vi "Parcial-Ascensor.vi"() -> ()   [LabVIEW 2018]
panel:
  out "PISO 4":bool
  out "PISO 3":bool
  out "PISO 2":bool
  out "PISO 1":bool
  in  "Ring":u16(ring)
  in  "Bajar4":bool
  in  "Bajar3":bool
  in  "Subir3":bool
  in  "Bajar2":bool
  in  "Subir2":bool
  in  "Subir1":bool
  out "4":bool
  out "3":bool
  out "2":bool
  out "1":bool
  out "P-der":dbl(slide) scale=0.0..10.0
  out "P-izq":dbl(slide)
  in  "Cerrar":bool
  in  "Abrir":bool
  out "Ascensor":bool
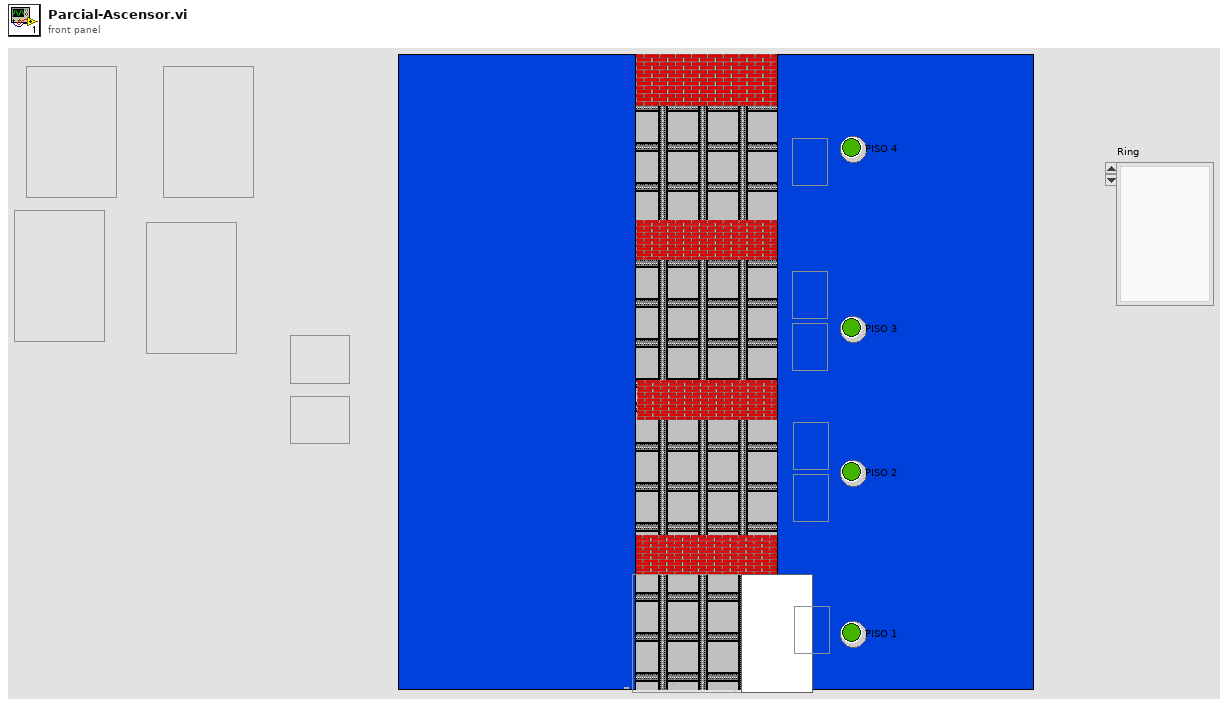
[diagram p1: front panel]
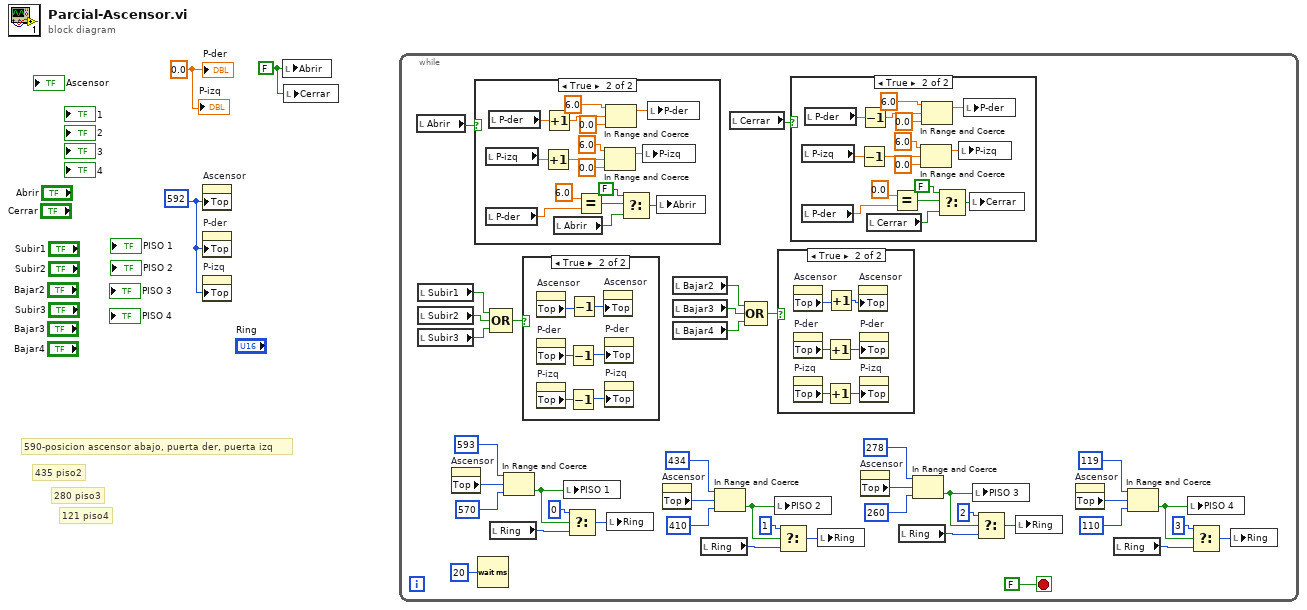
[diagram p0: block diagram]
diagram:
  w1 = 592 ("Position:Top")
  w3 = FALSE ("Abrir")
  w2 = 0.0 ("P-der")
  # "121 piso4"
  # "280 piso3"
  # "435 piso2"
  # "590-posicion ascensor abajo, puerta der, puerta izq"
  n1 = property on="Ascensor" class="Bool (strict)"("Top"=w1) -> ()  [unwired: 2 in, 2 out]
  n2 = property on="P-der" class="Slide (strict)"("Top"=w1) -> ()  [unwired: 2 in, 2 out]
  n3 = property on="P-izq" class="Slide (strict)"("Top"=w1) -> ()  [unwired: 2 in, 2 out]
  n4 = local write "Abrir"(w3) -> ()
  n5 = local write "Cerrar"(w3) -> ()
  n6 = while {
    stop <- FALSE stop-if-true
    n7 = local read "Abrir"() -> (w41:bool)
    n8 = local read "Subir1"() -> (w39:bool)
    n9 = local read "Subir2"() -> (w38:bool)
    n10 = local read "Subir3"() -> (w37:bool)
    n11 = property on="Ascensor" class="Bool (strict)"() -> ("Top"=w35:i32)  [unwired: 2 in, 2 out]
    n12 = case shown="True" w41 {
      frame False {
      }
      frame True {
        n13 = local read "P-izq"() -> (w87:dbl)
        n14 = local read "P-der"() -> (w72:dbl)
        n15 = local read "P-der"() -> (w86:dbl)
        n16 = Increment(x=w87) -> (x+1=w79:dbl)
        n17 = Increment(x=w86) -> (x+1=w85:dbl)
        n18 = local read "Abrir"() -> (w73:bool)
        n19 = Equal?(x=6.0, y=w72) -> (x = y?=w77:bool)
        n20 = In Range and Coerce(upper limit=6.0, x=w79, lower limit=0.0) -> (coerced(x)=w80:dbl)  [unwired: 1 out]
        n21 = In Range and Coerce(upper limit=6.0, x=w85, lower limit=0.0) -> (coerced(x)=w82:dbl)  [unwired: 1 out]
        n22 = Select(t=FALSE ("Abrir"), s=w77, f=w73) -> (s? t:f=w74:bool)
        n23 = local write "P-izq"(w80) -> ()
        n24 = local write "P-der"(w82) -> ()
        n25 = local write "Abrir"(w74) -> ()
      }
    }
    n26 = Wait (ms)(milliseconds to wait=u32 20) -> ()  [unwired: 1 out]
    n27 = Compound Arithmetic op=OR(w39, w38, w37) -> (w36:bool)
    n28 = local read "Ring"() -> (w31:u16)
    n29 = In Range and Coerce(upper limit=593 ("lower limit"), x=w35, lower limit=570 ("upper limit")) -> (In Range?=w34:bool)  [unwired: 1 out]
    n30 = case shown="True" w36 {
      frame False {
      }
      frame True {
        n31 = property on="Ascensor" class="Bool (strict)"() -> ("Top"=w55:i32)  [unwired: 2 in, 2 out]
        n32 = property on="P-der" class="Slide (strict)"() -> ("Top"=w53:i32)  [unwired: 2 in, 2 out]
        n33 = property on="P-izq" class="Slide (strict)"() -> ("Top"=w51:i32)  [unwired: 2 in, 2 out]
        n34 = Decrement(x=w53) -> (x-1=w52:i32)
        n35 = Decrement(x=w51) -> (x-1=w50:i32)
        n36 = Decrement(x=w55) -> (x-1=w54:i32)
        n37 = property on="Ascensor" class="Bool (strict)"("Top"=w54) -> ()  [unwired: 2 in, 2 out]
        n38 = property on="P-der" class="Slide (strict)"("Top"=w52) -> ()  [unwired: 2 in, 2 out]
        n39 = property on="P-izq" class="Slide (strict)"("Top"=w50) -> ()  [unwired: 2 in, 2 out]
      }
    }
    n40 = local write "PISO 1"(w34) -> ()
    n41 = Select(t=u16 0, s=w34, f=w31) -> (s? t:f=w33:u16)
    n42 = local write "Ring"(w33) -> ()
    n43 = property on="Ascensor" class="Bool (strict)"() -> ("Top"=w18:i32)  [unwired: 2 in, 2 out]
    n44 = local read "Bajar2"() -> (w25:bool)
    n45 = local read "Bajar3"() -> (w26:bool)
    n46 = local read "Bajar4"() -> (w27:bool)
    n47 = local read "Ring"() -> (w22:u16)
    n48 = In Range and Coerce(upper limit=434 ("lower limit"), x=w18, lower limit=410 ("upper limit")) -> (In Range?=w19:bool)  [unwired: 1 out]
    n49 = local read "Cerrar"() -> (w40:bool)
    n50 = Compound Arithmetic op=OR(w25, w26, w27) -> (w28:bool)
    n51 = local write "PISO 2"(w19) -> ()
    n52 = case shown="True" w28 {
      frame False {
      }
      frame True {
        n53 = property on="Ascensor" class="Bool (strict)"() -> ("Top"=w49:i32)  [unwired: 2 in, 2 out]
        n54 = property on="P-der" class="Slide (strict)"() -> ("Top"=w47:i32)  [unwired: 2 in, 2 out]
        n55 = property on="P-izq" class="Slide (strict)"() -> ("Top"=w45:i32)  [unwired: 2 in, 2 out]
        n56 = Increment(x=w47) -> (x+1=w46:i32)
        n57 = Increment(x=w45) -> (x+1=w44:i32)
        n58 = Increment(x=w49) -> (x+1=w48:i32)
        n59 = property on="Ascensor" class="Bool (strict)"("Top"=w48) -> ()  [unwired: 2 in, 2 out]
        n60 = property on="P-der" class="Slide (strict)"("Top"=w46) -> ()  [unwired: 2 in, 2 out]
        n61 = property on="P-izq" class="Slide (strict)"("Top"=w44) -> ()  [unwired: 2 in, 2 out]
      }
    }
    n62 = Select(t=u16 1, s=w19, f=w22) -> (s? t:f=w20:u16)
    n63 = case shown="True" w40 {
      frame False {
      }
      frame True {
        n64 = local read "P-izq"() -> (w71:dbl)
        n65 = local read "P-der"() -> (w56:dbl)
        n66 = local read "P-der"() -> (w70:dbl)
        n67 = Decrement(x=w71) -> (x-1=w63:dbl)
        n68 = Decrement(x=w70) -> (x-1=w69:dbl)
        n69 = local read "Cerrar"() -> (w57:bool)
        n70 = Equal?(x=0.0, y=w56) -> (x = y?=w61:bool)
        n71 = In Range and Coerce(upper limit=6.0, x=w63, lower limit=0.0) -> (coerced(x)=w64:dbl)  [unwired: 1 out]
        n72 = In Range and Coerce(upper limit=6.0, x=w69, lower limit=0.0) -> (coerced(x)=w66:dbl)  [unwired: 1 out]
        n73 = Select(t=FALSE ("Abrir"), s=w61, f=w57) -> (s? t:f=w58:bool)
        n74 = local write "P-izq"(w64) -> ()
        n75 = local write "P-der"(w66) -> ()
        n76 = local write "Cerrar"(w58) -> ()
      }
    }
    n77 = local write "Ring"(w20) -> ()
    n78 = property on="Ascensor" class="Bool (strict)"() -> ("Top"=w17:i32)  [unwired: 2 in, 2 out]
    n79 = local read "Ring"() -> (w13:u16)
    n80 = In Range and Coerce(upper limit=278 ("lower limit"), x=w17, lower limit=260 ("upper limit")) -> (In Range?=w16:bool)  [unwired: 1 out]
    n81 = local write "PISO 3"(w16) -> ()
    n82 = Select(t=u16 2, s=w16, f=w13) -> (s? t:f=w15:u16)
    n83 = local write "Ring"(w15) -> ()
    n84 = property on="Ascensor" class="Bool (strict)"() -> ("Top"=w4:i32)  [unwired: 2 in, 2 out]
    n85 = local read "Ring"() -> (w8:u16)
    n86 = In Range and Coerce(upper limit=119 ("lower limit"), x=w4, lower limit=110 ("upper limit")) -> (In Range?=w5:bool)  [unwired: 1 out]
    n87 = local write "PISO 4"(w5) -> ()
    n88 = Select(t=u16 3, s=w5, f=w8) -> (s? t:f=w6:u16)
    n89 = local write "Ring"(w6) -> ()
  }
  "P-izq" <- w2
  "P-der" <- w2
